vi "Drive_Set.vi"   [LabVIEW 2020]
uses:
  Globals/Drive_Globals.vi
  Drive_Control_States.ctl
  Robot Global Data.vi
  <vilib>/Rock Robotics/WPI/DriverStation/WPI_DriverStationRobotMode2.ctl
  Drive_Orientation_States.ctl
  Drive_Cluster.ctl
  Systems/Shooter/Determiner/Shooter_Globals.vi
  Systems/Shooter/Determiner/Shooter_Control_States.ctl
panel:
  # "e"
types:
  T1 = typedef "Shooter_Control_States.ctl" = enum16{"No-Op", "Limelight_Shooting", "Shoot_From_Pose", "Test", "Command_ShootFromPose", "Command_Shoot", "Turret_Cowl_Zero", "Manual", "Puke-Op", "Auto_Track"}
  T2 = typedef "Drive_Cluster.ctl" = cluster{"Control_State":T3, "Vertical_Throttle":dbl, "Lateral_Throttle":dbl, "Rotational_Throttle":dbl, "Strafe_In_Deadband":bool, "Rotation_In_Deadband":bool, "Orientation_State":T4, "Parameters":dbl[], "Step":i32, "Auto_Notifier":refnum<notifier>, "PathName":string}
  T3 = typedef "Drive_Control_States.ctl" = enum16{"No-Op", "Manual_Control", "Command_DriveDistanceAtAngle", "Command_DrivePath", "Command_SetRobotPose", "Command_Rotate", "Go_To_X"}
  T4 = typedef "Drive_Orientation_States.ctl" = enum16{"Robot-Oriented", "Field-Oriented"}
  T5 = typedef "WPI_DriverStationRobotMode2.ctl" = enum16{"Autonomous Disabled", "Autonomous Enabled", "Teleop Disabled", "Teleop Enabled", "Disconnected", "Finish", "Test Disabled", "Test Enabled", "Emergency Stopped"}
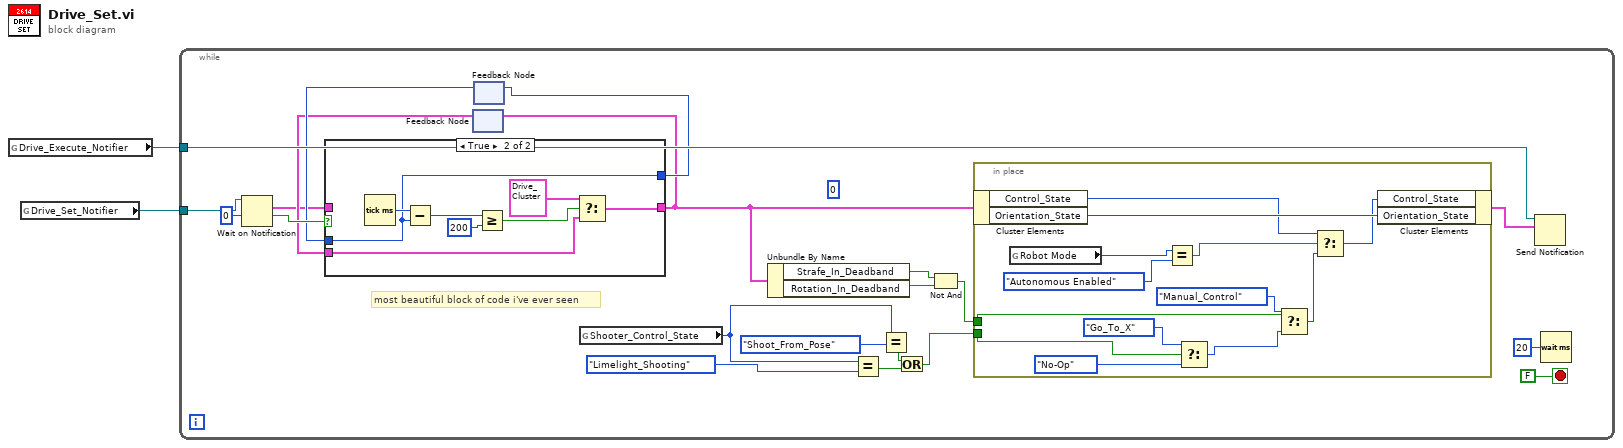
[diagram p0: block diagram]
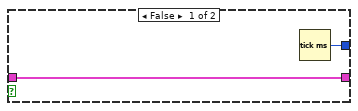
[diagram p2: hidden frame]
diagram:
  n1 = global read "Drive_Globals.vi" "Drive_Execute_Notifier"() -> (w2:refnum<notifier>)
  n2 = global read "Drive_Globals.vi" "Drive_Set_Notifier"() -> (w1:refnum<notifier>)
  n3 = while {
    tunnel: w2 -> [w20]
    tunnel: w1 -> [w21]
    stop <- FALSE stop-if-true
    (unwired) 0 ("timeout in ms (-1)")
    # "most beautiful block of code i've ever seen"
    n4 = Wait on Notification(notifier=w21, timeout in ms (-1)=0) -> (notification=w10:T2, timed out?=w14:bool)  [unwired: 2 in, 2 out]
    n5 = feedback #1() -> (w11:T2)  [unwired: 1 in]
    n6 = feedback #2() -> (w12:u32)  [unwired: 1 in]
    n7 = case shown="True" w14 {
      tunnel: w10 -> [w25 _]
      tunnel: [w25 w33] -> w9
      tunnel: w11 -> [_ w32]
      tunnel: [w24 w30] -> w13
      tunnel: w12 -> [_ w30]
      frame False {
        n8 = Tick Count (ms)() -> (millisecond timer value=w24:u32)
      }
      frame True {
        n9 = Tick Count (ms)() -> (millisecond timer value=w31:u32)
        n10 = Subtract(x=w31, y=w30) -> (x-y=w28:u32)
        n11 = Greater Or Equal?(x=w28, y=u32 200) -> (x >= y?=w29:bool)
        n12 = Select(t=T2 {"Control_State"=enum."Manual_Control", "Vertical_Throttle"=0.0, "Lateral_Throttle"=0.0, "Rotational_Throttle"=0.0, "Strafe_In_Deadband"=FALSE, "Rotation_In_Deadband"=FALSE, "Orientation_State"=enum."Robot-Oriented", "Parameters"=[], "Step"=0, "Auto_Notifier"=refnum, "PathName"=""} ("Cluster"), s=w29, f=w32) -> (s? t:f=w33:T2)
      }
    }
    n13 = feedback-in #1(w9) -> ()
    n14 = feedback-in #2(w13) -> ()
    n15 = global read "Shooter_Globals.vi" "Shooter_Control_State"() -> (w5:T1)
    n16 = Unbundle By Name(w9) -> ("Strafe_In_Deadband"=w17:bool, "Rotation_In_Deadband"=w16:bool)
    n17 = Equal?(x=w5, y=Shooter_Control_States."Limelight_Shooting") -> (x = y?=w7:bool)
    n18 = Equal?(x=w5, y=Shooter_Control_States."Shoot_From_Pose") -> (x = y?=w6:bool)
    n19 = Or(x=w6, y=w7) -> (x .or. y?=w3:bool)
    n20 = Not And(1:w16, 2:w17) -> (0:w15:bool)
    n21 = in-place {
      in-place-border: w15 -> [w38]
      in-place-border: w3 -> [w37]
      n22 = in-place-cluster #3(w9) -> ("Control_State"=w41:T3, "Orientation_State"=w46:T4)
      n23 = global read "Robot Global Data.vi" "Robot Mode"() -> (w44:T5)
      n24 = Equal?(x=w44, y=WPI_DriverStationRobotMode2."Autonomous Enabled" ("Robot Mode")) -> (x = y?=w43:bool)
      n25 = Select(t=Drive_Control_States."Go_To_X" ("Control_State"), s=w37, f=Drive_Control_States."No-Op" ("Control_State")) -> (s? t:f=w34:T3)
      n26 = Select(t=Drive_Control_States."Manual_Control" ("Control_State"), s=w38, f=w34) -> (s? t:f=w39:T3)
      n27 = Select(t=w41, s=w43, f=w39) -> (s? t:f=w42:T3)
      n28 = in-place-cluster #3("Control_State"=w42, "Orientation_State"=w46) -> (w19:T2)
    }
    n29 = Send Notification(notification=w19, notifier=w20) -> ()  [unwired: 1 in, 2 out]
    n30 = Wait (ms)(milliseconds to wait=u32 20) -> ()  [unwired: 1 out]
  }
